vi "Adjust Bounds.vi"(6 "Control Ref Cluster":T1, 8 "error in (no error)":errorcluster) -> (0 "error out":errorcluster)   [LabVIEW 2017, in "2D Plot.lvclass"]
uses:
  <vilib>/Math Plots/2D Math Plots/2D Plot/2D Plot/2D Plot.lvclass
  <vilib>/Math Plots/2D Math Plots/2D Plot/Action String/2DMathPlot Ctrl Act Cluster.ctl
  <vilib>/Math Plots/2D Math Plots/2D Plot/Action String/2DMathPlot State Class.ctl
  <vilib>/Math Plots/Plot Private Lib/NI_Math Plot Private Lib.lvlib
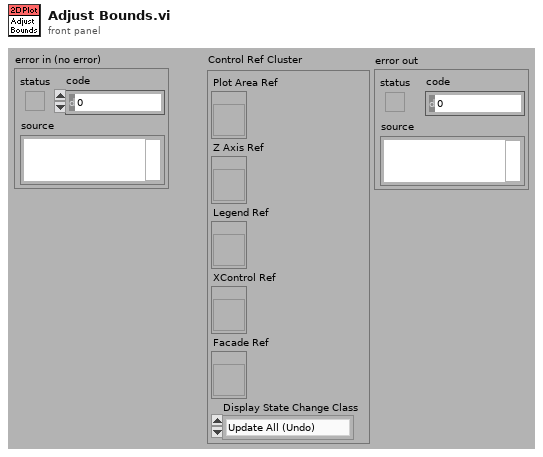
[diagram p1: front panel]
types:
  T1 = typedef "2DMathPlot Ctrl Act Cluster.ctl" = cluster{"Plot Area Ref":refnum<vi>, "Z Axis Ref":refnum<vi>, "Legend Ref":refnum<vi>, "XControl Ref":refnum<vi>, "Facade Ref":refnum<vi>, "Display State Change Class":T2}
  T2 = typedef "2DMathPlot State Class.ctl" = enum16{"Update All (Undo)", "Update General", "Update Appearance", "Update Format", "Update Scale", "Update Marker", "Update Cursor", "None"}
  T3 = enum16{"No Scaling", "Scale All Objects", "Scale Single Object"}
  T4 = typedef "LVBoundsTypeDef.ctl" = cluster{"Width":u32, "Height":u32}
  T5 = typedef "LVRectTypeDef.ctl" = cluster{"Left":i16, "Top":i16, "Right":i16, "Bottom":i16}
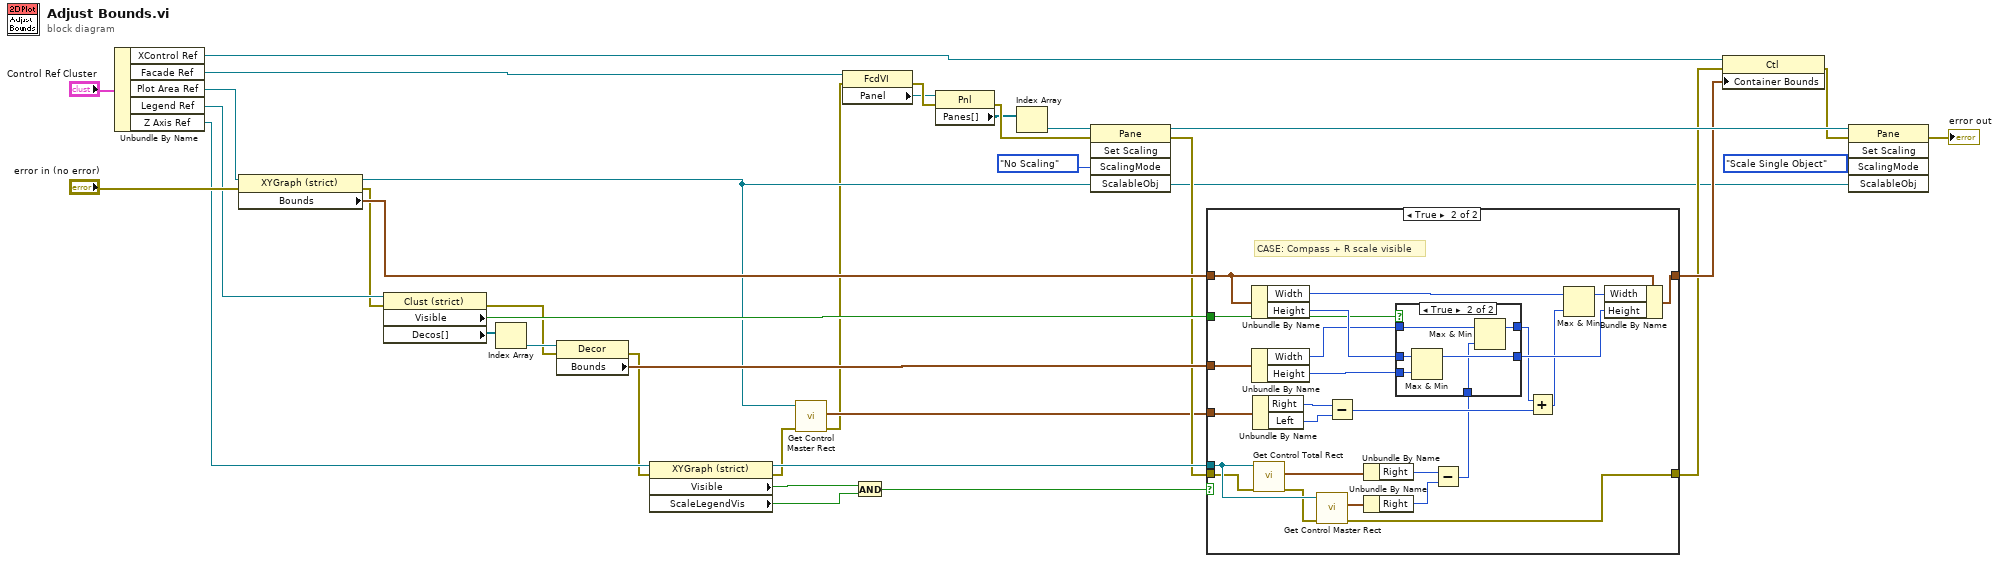
[diagram p0: block diagram]
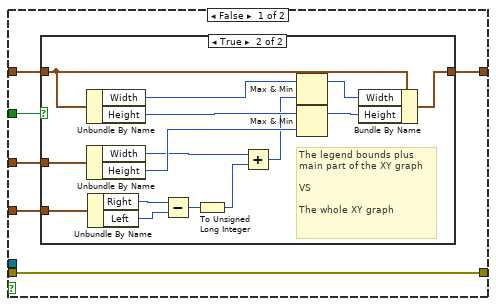
[diagram p2: hidden frame]
diagram:
  n1 = Unbundle By Name("Control Ref Cluster") -> ("XControl Ref"=w24:refnum<vi>, "Facade Ref"=w29:refnum<vi>, "Plot Area Ref"=w27:refnum<vi>, "Legend Ref"=w21:refnum<vi>, "Z Axis Ref"=w12:refnum<vi>)
  n2 = property class="XYGraph (strict)"(reference=w27, error in="error in (no error)") -> (reference out=w3:refnum<vi>, error out=w18:errorcluster, "Bounds"=w20:T4)
  n3 = property class="Clust (strict)"(reference=w21, error in=w18) -> (error out=w13:errorcluster, "Visible"=w17:bool, "Decos[]"=w16:refnum<vi>[])  [unwired: 1 out]
  n4 = Index Array(array=w16) -> (element=w15:refnum<vi>)  [unwired: 1 in]
  n5 = property class="Decor"(reference=w15, error in=w13) -> (error out=w7:errorcluster, "Bounds"=w14:T4)  [unwired: 1 out]
  n6 = property class="XYGraph (strict)"(reference=w12, error in=w7) -> (reference out=w8:refnum<vi>, error out=w2:errorcluster, "Visible"=w11:bool, "ScaleLegendVis"=w10:bool)
  n7 = call <vilib>:"Get Control Master Rect.vi"("error in (no error)"=w2, "reference"=w3) -> ("error out"=w1:errorcluster, "Master Bounds Rect"=w4:T5)  [unwired: 8 out]
  n8 = property class="FcdVI"(reference=w29, error in=w1) -> (error out=w34:errorcluster, "Panel"=w30:refnum<vi>)  [unwired: 1 out]
  n9 = And(x=w11, y=w10) -> (x .and. y?=w9:bool)
  n10 = property class="Pnl"(reference=w30, error in=w34) -> (error out=w35:errorcluster, "Panes[]"=w31:refnum<vi>[])  [unwired: 1 out]
  n11 = Index Array(array=w31) -> (element=w32:refnum<vi>)  [unwired: 1 in]
  n12 = invoke class="Pane" method="Set Scaling"(reference=w32, error in=w35, "ScalingMode"=T3."No Scaling" ("Scaling Mode"), "ScalableObj"=w3) -> (reference out=w25:refnum<vi>, error out=w6:errorcluster)  [unwired: 1 in, 3 out]
  n13 = case shown="True" w9 {
    tunnel: w20 -> [w42 w76]
    tunnel: [w41 w83] -> w19
    tunnel: w17 -> [w40 w70]
    tunnel: w14 -> [w39 w74]
    tunnel: w4 -> [w38 w78]
    tunnel: w8 -> [_ w69]
    tunnel: w6 -> [w37 w66]
    tunnel: [w37 w64] -> w5
    frame False {
      n14 = case shown="True" w40 {
        tunnel: w42 -> [w43 w57]
        tunnel: [w43 w56] -> w41
        tunnel: w39 -> [_ w58]
        tunnel: w38 -> [_ w51]
        frame False {
          # "If the customized legend is invisible,\nXControl bounds is same with XY graph\n bounds"
        }
        frame True {
          # "The legend bounds plus \nmain part of the XY graph\n\nVS\n\nThe whole XY graph"
          n15 = Unbundle By Name(w57) -> ("Width"=w46:u32, "Height"=w54:u32)
          n16 = Unbundle By Name(w58) -> ("Width"=w52:u32, "Height"=w55:u32)
          n17 = Unbundle By Name(w51) -> ("Right"=w50:i16, "Left"=w49:i16)
          n18 = Subtract(x=w50, y=w49) -> (x-y=w48:i16)
          n19 = To Unsigned Long Integer(number=w48) -> (unsigned 32bit integer=w47:u32)
          n20 = Add(x=w52, y=w47) -> (x+y=w45:u32)
          n21 = Max & Min(x=w46, y=w45) -> (max(x,y)=w44:u32)  [unwired: 1 out]
          n22 = Max & Min(x=w54, y=w55) -> (max(x,y)=w53:u32)  [unwired: 1 out]
          n23 = Bundle By Name(cluster=w57, "Width"=w44, "Height"=w53) -> (w56:T4)
        }
      }
    }
    frame True {
      # "CASE: Compass + R scale visible"
      n24 = Unbundle By Name(w76) -> ("Width"=w63:u32, "Height"=w73:u32)
      n25 = Unbundle By Name(w74) -> ("Width"=w61:u32, "Height"=w72:u32)
      n26 = Unbundle By Name(w78) -> ("Right"=w80:i16, "Left"=w79:i16)
      n27 = call <vilib>:"Get Control Total Rect.vi"("error in (no error)"=w66, "reference"=w69) -> ("error out"=w65:errorcluster, "Total Bounds Rect"=w68:T5)  [unwired: 8 out]
      n28 = call <vilib>:"Get Control Master Rect.vi"("error in (no error)"=w65, "reference"=w69) -> ("error out"=w64:errorcluster, "Master Bounds Rect"=w67:T5)  [unwired: 8 out]
      n29 = Subtract(x=w80, y=w79) -> (x-y=w77:i16)
      n30 = Unbundle By Name(w68) -> ("Right"=w82:i16)
      n31 = Unbundle By Name(w67) -> ("Right"=w81:i16)
      n32 = Subtract(x=w82, y=w81) -> (x-y=w60:i16)
      n33 = case shown="True" w70 {
        tunnel: w73 -> [w85 w91]
        tunnel: w72 -> [_ w90]
        tunnel: [w85 w89] -> w71
        tunnel: w61 -> [_ w88]
        tunnel: w60 -> [w84 w87]
        tunnel: [w84 w86] -> w59
        frame False {
        }
        frame True {
          n34 = Max & Min(x=w91, y=w90) -> (max(x,y)=w89:u32)  [unwired: 1 out]
          n35 = Max & Min(x=w88, y=w87) -> (max(x,y)=w86:u32)  [unwired: 1 out]
        }
      }
      n36 = Add(x=w59, y=w77) -> (x+y=w62:u32)
      n37 = Max & Min(x=w63, y=w62) -> (max(x,y)=w75:u32)  [unwired: 1 out]
      n38 = Bundle By Name(cluster=w76, "Width"=w75, "Height"=w71) -> (w83:T4)
    }
  }
  n39 = property class="Ctl"(reference=w24, error in=w5, "Container Bounds"=w19) -> (error out=w23:errorcluster)  [unwired: 1 out]
  n40 = invoke class="Pane" method="Set Scaling"(reference=w25, error in=w23, "ScalingMode"=T3."Scale Single Object" ("Scaling Mode"), "ScalableObj"=w3) -> (error out=→"error out":errorcluster)  [unwired: 1 in, 4 out]
